vi "filter trigger.vi"(8 "error in":errorcluster, 10 "Line(s)":tag="Dev1/port0/line0:7", 11 "filter time(s)*10":i32=100) -> (0 "error out":errorcluster)   [LabVIEW 2018]
uses:
  <vilib>/Utility/error.llb/DialogType.ctl
  <vilib>/DAQmx/write.llb/DAQmx Write (Digital 1D U32 1Chan NSamp).vi
  <vilib>/DAQmx/create/channels.llb/DAQmx Create Channel (DO-Digital Output).vi
  <vilib>/DAQmx/configure/timing.llb/DAQmx Timing (Sample Clock).vi
  <vilib>/DAQmx/miscellaneous.llb/DAQmx Fill In Error Info.vi
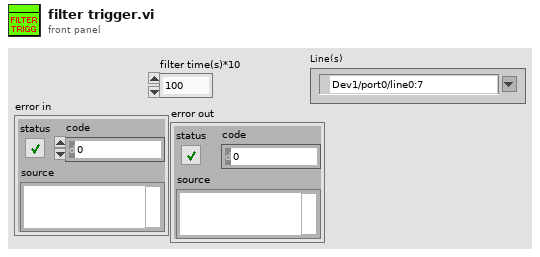
[diagram p1: front panel]
types:
  T1 = typedef "DialogType.ctl" = u16
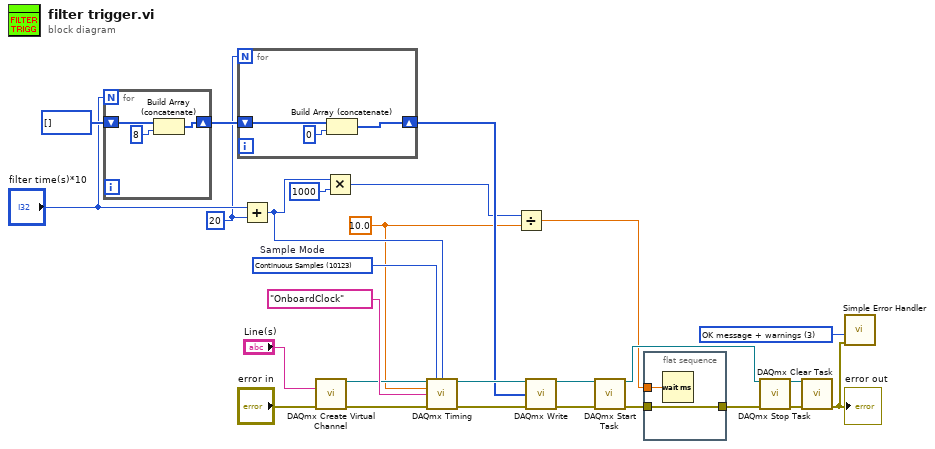
[diagram p0: block diagram]
diagram:
  w8 = 20
  w4 = 10.0 ("Sample Rate")
  w20 = T1 3 items=["no dialog", "OK message", "continue or stop message", "OK message + warnings", "continue/stop + warnings"] ("type of dialog (OK msg:1)")
  w24 = 10123 items=["Finite Samples"=10178, "Continuous Samples"=10123, "Hardware Timed Single Point"=12522]  # Sample Mode
  n1 = for {
    N: "filter time(s)*10" -> [_]
    shift-right: [w28] -> w11
    shift-left: i32[] [] -> [w30]
    n2 = Build Array (concatenate)(w30, 8 ("element")) -> (w28:i32[])
  }
  n3 = for {
    N: w8 -> [_]
    shift-right: [w31] -> w10
    shift-left: w11 -> [w33]
    n4 = Build Array (concatenate)(w33, 0 ("element")) -> (w31:i32[])
  }
  n5 = Add(x="filter time(s)*10", y=w8) -> (x+y=w7:i32)
  n6 = call-poly <vilib>:"DAQmx Create Virtual Channel.vi"("lines"="Line(s)", "error in"="error in") -> ("task out"=w26:refnum<k21>, "error out"=w25:errorcluster)  [unwired: 12 in]
  n7 = Multiply(x=w7, y=1000) -> (x*y=w5:i32)
  n8 = call-poly <vilib>:"DAQmx Timing.vi"("task/channels in"=w26, "sample mode"=w24, "samples per channel"=w7, "rate"=w4, "source"=tag "OnboardClock" ("Sample Clock Source"), "error in"=w25) -> ("task out"=w18:refnum<k21>, "error out"=w19:errorcluster)  [unwired: 8 in]
  n9 = Divide(x=w5, y=w4) -> (x/y=w3:dbl)
  n10 = call-poly <vilib>:"DAQmx Write.vi"("task/channels in"=w18, "data"=w10, "error in"=w19) -> ("task out"=w16:refnum<k21>, "error out"=w13:errorcluster)  [unwired: 10 in, 1 out]
  n11 = call <vilib>:"DAQmx Start Task.vi"("task/channels in"=w16, "error in"=w13) -> ("task out"=w17:refnum<k21>, "error out"=w15:errorcluster)  [unwired: 12 in]
  n12 = flat-sequence {
    tunnel: w15 -> [w35]
    tunnel: [w35] -> w14
    tunnel: w3 -> [w34]
    frame #0 {
      n13 = Wait (ms)(milliseconds to wait=w34) -> ()  [unwired: 1 out]
    }
  }
  n14 = call <vilib>:"DAQmx Stop Task.vi"("task/channels in"=w17, "error in"=w14) -> ("task out"=w22:refnum<k21>, "error out"=w21:errorcluster)  [unwired: 12 in]
  n15 = call <vilib>:"DAQmx Clear Task.vi"("task in"=w22, "error in"=w21) -> ("error out"=w1:errorcluster)  [unwired: 13 in]
  "error out" <- w1
  n16 = call <vilib>:"Simple Error Handler.vi"("type of dialog (OK msg:1)"=w20, "error in (no error)"=w1) -> ()  [unwired: 3 in, 5 out]
